vi "Cutie de viteze.vi"() -> ()   [LabVIEW 2020]
panel:
  in  "Start - Stop":bool
  out "Rpm":dbl
  out "Km/h":dbl
  in  "Treapta Sus":dbl
  out "Treapta Viteza":dbl
  out "Viteza":dbl(knob) scale=0.0..300.0
  out "Turatie":dbl(knob) scale=0.0..6000.0
  out "Up":bool
  in  "Pedala frana":dbl(slide) scale=0.0..100.0
  in  "Pedala Acceleratie":dbl(slide) scale=0.0..100.0
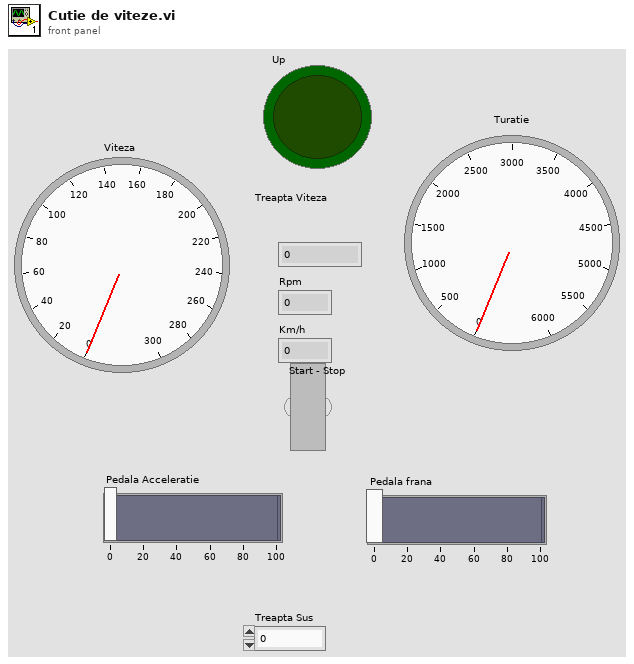
[diagram p1: front panel]
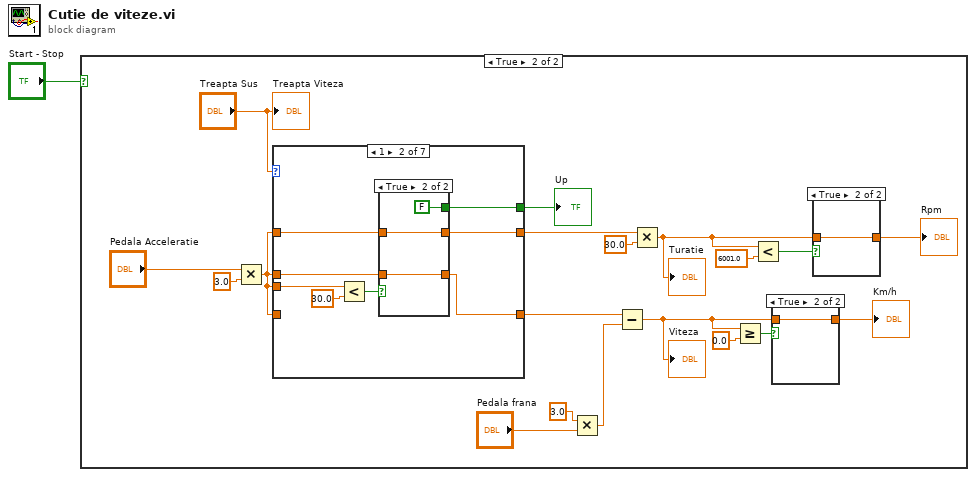
[diagram p0: block diagram]
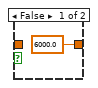
[diagram p3: hidden frame]
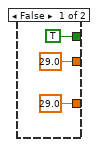
[diagram p6: hidden frame]
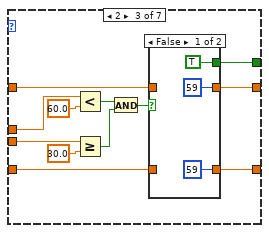
[diagram p7: hidden frame]
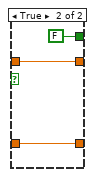
[diagram p8: hidden frame]
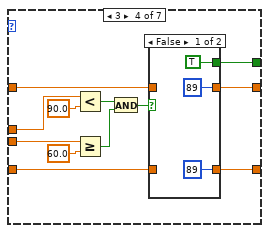
[diagram p9: hidden frame]
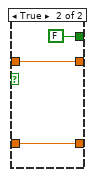
[diagram p10: hidden frame]
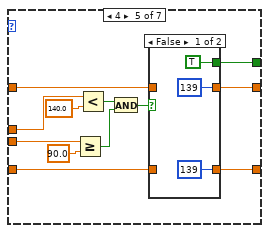
[diagram p11: hidden frame]
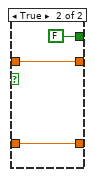
[diagram p12: hidden frame]
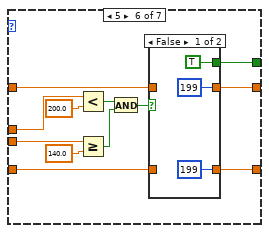
[diagram p13: hidden frame]
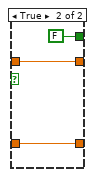
[diagram p14: hidden frame]
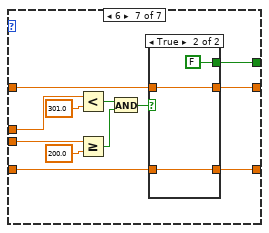
[diagram p15: hidden frame]
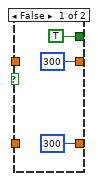
[diagram p16: hidden frame]
diagram:
  n1 = case shown="True" "Start - Stop" {
    frame False {
    }
    frame True {
      n2 = Multiply(x="Pedala Acceleratie", y=3.0) -> (x*y=w6:dbl)
      n3 = case shown="1" "Treapta Sus" {
        tunnel: w6 -> [_ w29 w46 w61 w79 w97 w115]
        tunnel: w6 -> [_ w28 w48 w62 w80 w98 w116]
        tunnel: [_ w27 w41 w59 w77 w95 w113] -> w17
        tunnel: w6 -> [_ _ w42 w60 w78 w96 w114]
        tunnel: w6 -> [_ w26 w39 w58 w75 w93 w111]
        tunnel: [_ w25 w40 w57 w76 w94 w112] -> w19
        tunnel: [_ w24 w38 w56 w74 w92 w110] -> w18
        frame 0, Default {
        }
        frame 1 {
          n4 = Less?(x=w29, y=30.0) -> (x < y?=w30:bool)
          n5 = case shown="True" w30 {
            tunnel: w28 -> [_ w37]
            tunnel: [29.0 ("Pedala Acceleratie") w37] -> w27
            tunnel: w26 -> [_ w36]
            tunnel: [29.0 ("Pedala Acceleratie") w36] -> w25
            tunnel: [TRUE FALSE] -> w24
            frame False {
            }
            frame True {
            }
          }
        }
        frame 2 {
          n6 = Less?(x=w48, y=60.0) -> (x < y?=w45:bool)
          n7 = Greater Or Equal?(x=w46, y=30.0) -> (x >= y?=w44:bool)
          n8 = And(x=w45, y=w44) -> (x .and. y?=w43:bool)
          n9 = case shown="False" w43 {
            tunnel: w42 -> [_ w55]
            tunnel: [59 w55] -> w41
            tunnel: [59 w54] -> w40
            tunnel: w39 -> [_ w54]
            tunnel: [TRUE FALSE] -> w38
            frame False {
            }
            frame True {
            }
          }
        }
        frame 3 {
          n10 = Less?(x=w62, y=90.0) -> (x < y?=w65:bool)
          n11 = Greater Or Equal?(x=w61, y=60.0) -> (x >= y?=w64:bool)
          n12 = And(x=w65, y=w64) -> (x .and. y?=w63:bool)
          n13 = case shown="False" w63 {
            tunnel: w60 -> [_ w73]
            tunnel: [89 w73] -> w59
            tunnel: w58 -> [_ w72]
            tunnel: [89 w72] -> w57
            tunnel: [TRUE FALSE] -> w56
            frame False {
            }
            frame True {
            }
          }
        }
        frame 4 {
          n14 = Greater Or Equal?(x=w79, y=90.0) -> (x >= y?=w82:bool)
          n15 = Less?(x=w80, y=140.0) -> (x < y?=w83:bool)
          n16 = And(x=w83, y=w82) -> (x .and. y?=w81:bool)
          n17 = case shown="False" w81 {
            tunnel: w78 -> [_ w91]
            tunnel: [139 w91] -> w77
            tunnel: [139 w90] -> w76
            tunnel: w75 -> [_ w90]
            tunnel: [TRUE FALSE] -> w74
            frame False {
            }
            frame True {
            }
          }
        }
        frame 5 {
          n18 = Less?(x=w98, y=200.0) -> (x < y?=w101:bool)
          n19 = Greater Or Equal?(x=w97, y=140.0) -> (x >= y?=w100:bool)
          n20 = And(x=w101, y=w100) -> (x .and. y?=w99:bool)
          n21 = case shown="False" w99 {
            tunnel: w96 -> [_ w109]
            tunnel: [199 w109] -> w95
            tunnel: [199 w108] -> w94
            tunnel: w93 -> [_ w108]
            tunnel: [TRUE FALSE] -> w92
            frame False {
            }
            frame True {
            }
          }
        }
        frame 6 {
          n22 = Less?(x=w116, y=301.0) -> (x < y?=w119:bool)
          n23 = Greater Or Equal?(x=w115, y=200.0) -> (x >= y?=w118:bool)
          n24 = And(x=w119, y=w118) -> (x .and. y?=w117:bool)
          n25 = case shown="True" w117 {
            tunnel: w114 -> [_ w127]
            tunnel: [300 w127] -> w113
            tunnel: [300 w126] -> w112
            tunnel: w111 -> [_ w126]
            tunnel: [TRUE FALSE] -> w110
            frame False {
            }
            frame True {
            }
          }
        }
      }
      "Up" <- w18
      n26 = Multiply(x=3.0 ("x*y"), y="Pedala frana") -> (x*y=w11:dbl)
      n27 = Subtract(x=w17, y=w11) -> (x-y=w13:dbl)
      "Viteza" <- w13
      n28 = Multiply(x=w19, y=30.0) -> (x*y=w3:dbl)
      "Turatie" <- w3
      n29 = Greater Or Equal?(x=w13, y=0.0) -> (x >= y?=w14:bool)
      n30 = Less?(x=w3, y=6001.0) -> (x < y?=w4:bool)
      n31 = case shown="True" w14 {
        tunnel: w13 -> [_ w23]
        tunnel: [_ w23] -> w12
        frame False {
        }
        frame True {
        }
      }
      "Km/h" <- w12
      n32 = case shown="True" w4 {
        tunnel: w3 -> [_ w22]
        tunnel: [6000.0 w22] -> w2
        frame False {
        }
        frame True {
        }
      }
      "Rpm" <- w2
      "Treapta Viteza" <- "Treapta Sus"
    }
  }
